vi "ScratchImage.vi"() -> ()   [LabVIEW 2020]
uses:
  <vilib>/Analysis/baseanly.llb/Mean (DBL).vi
  <vilib>/Analysis/NI_AALBase.lvlib
panel:
  in  "Save to Files":bool
  in  "Path":path
  out "height":dbl
  out "width":dbl
  out "y":dbl format="%0.2f"
  out "x":dbl format="%0.2f"
  out "new picture":picture
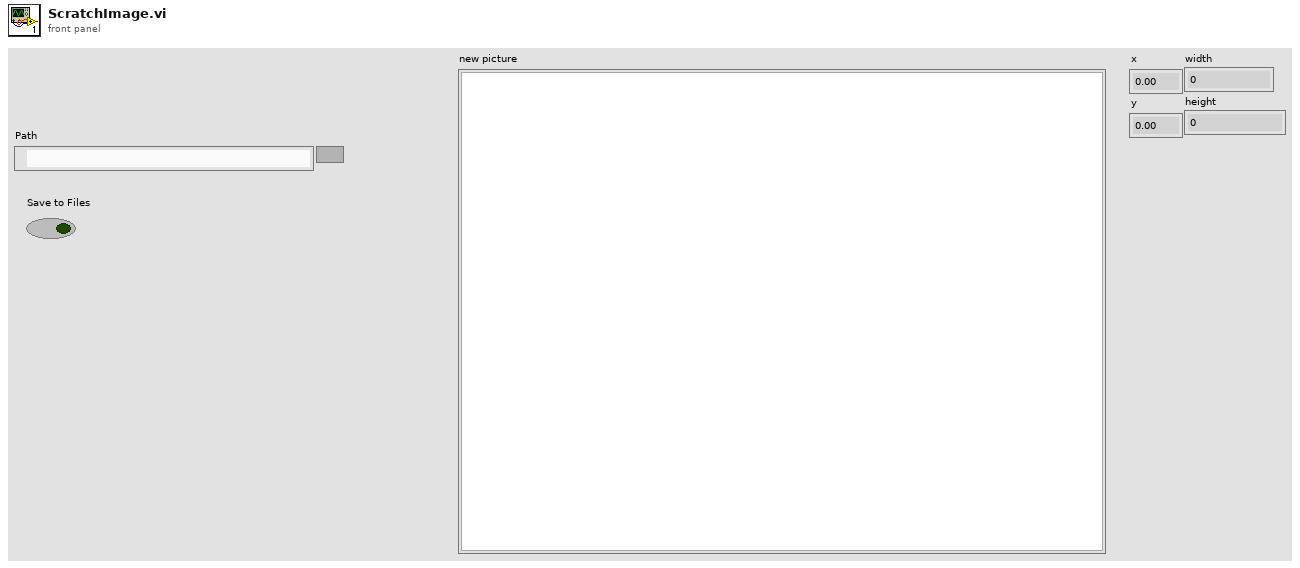
[diagram p1: front panel]
types:
  T1 = enum16{"open", "replace", "create", "open or create", "replace or create", "replace or create with confirmation"}
  T2 = cluster{"Width":u16, "Style":enum32{"Solid", "Dash", "Dot", "DashDot", "DashDotDot"}}
  T3 = enum32{"Solid", "Dash", "Dot", "DashDot", "DashDotDot"}
  T4 = typedef "imagedata.ctl" = cluster{"image type":i32, "image depth":i32, "image":u8[], "mask":u8[], "colors":u32[], "Rectangle":cluster{"left":i16, "top":i16, "right":i16, "bottom":i16}}
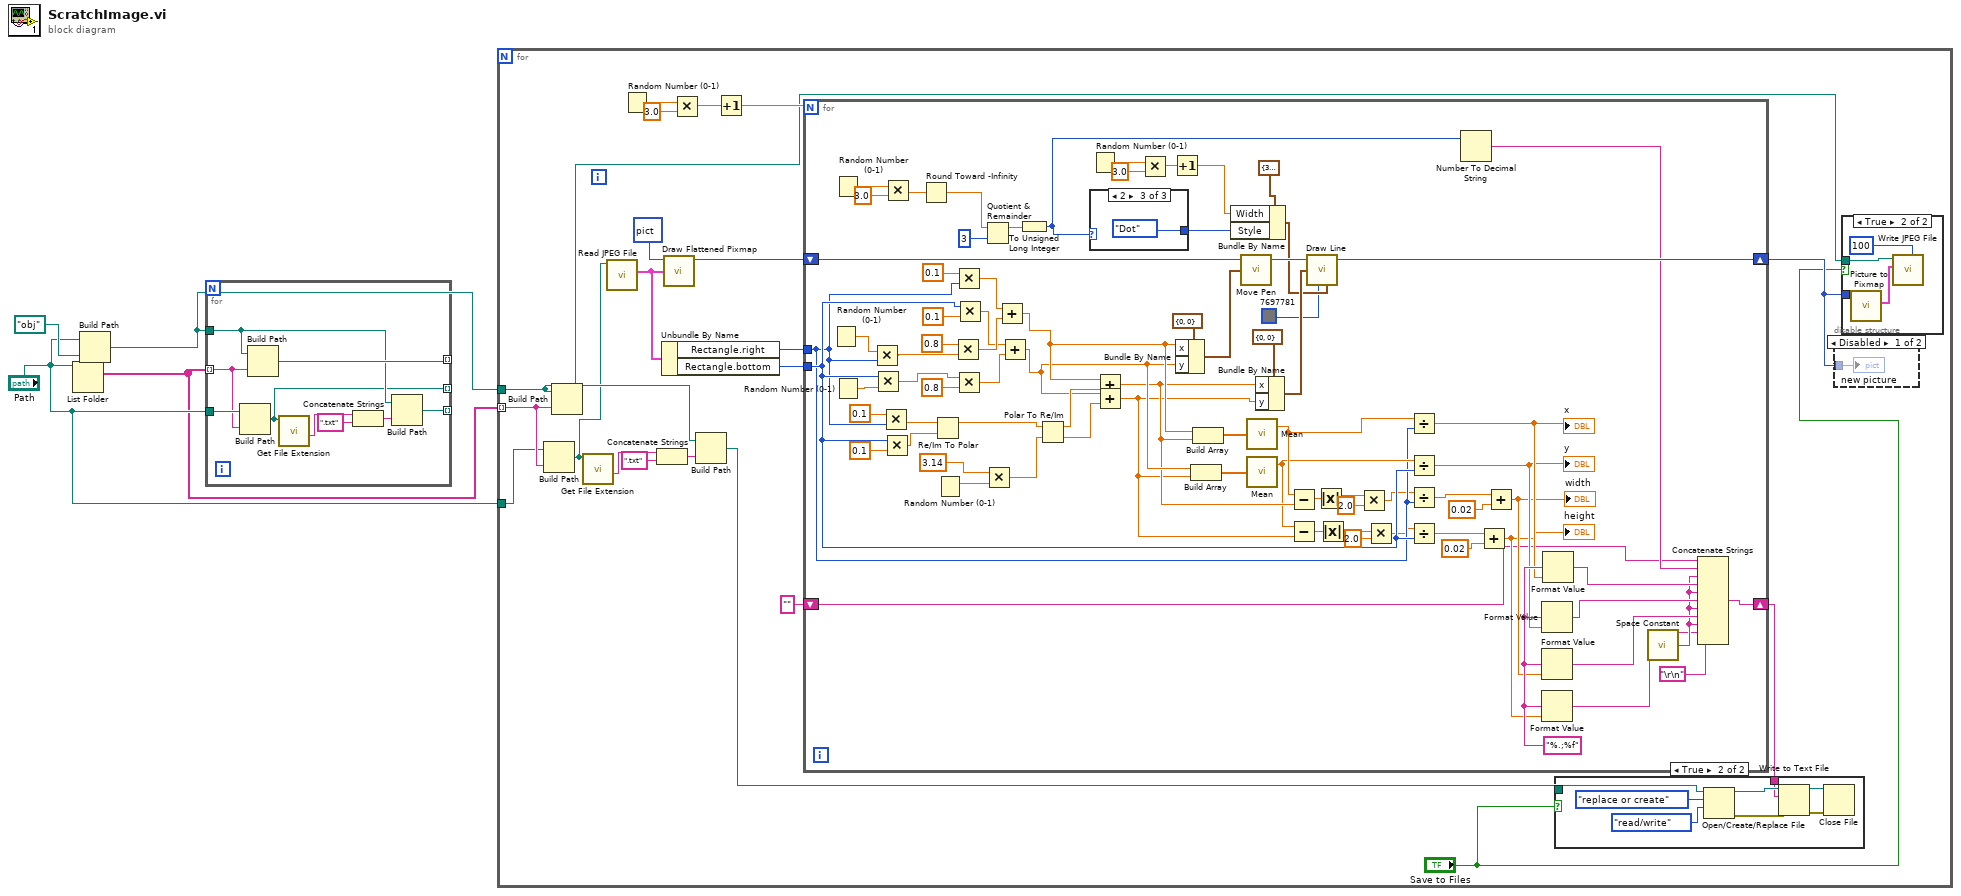
[diagram p0: block diagram]
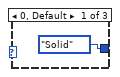
[diagram p5: hidden frame]
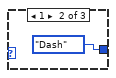
[diagram p6: hidden frame]
diagram:
  n1 = List Folder(path="Path") -> (filenames=w1:string[])  [unwired: 3 in, 3 out]
  n2 = Build Path(base path="Path", name or relative path=path "obj") -> (appended path=w3:path)
  n3 = for {
    tunnel: w1 -> [w11] mode=indexing
    tunnel: w3 -> [w10]
    tunnel: [w13] -> _ mode=indexing
    tunnel: "Path" -> [w12]
    tunnel: [w6] -> _ mode=indexing
    tunnel: [w5] -> _ mode=indexing
    n4 = Build Path(base path=w12, name or relative path=w11) -> (appended path=w5:path)
    n5 = Build Path(base path=w10, name or relative path=w11) -> (appended path=w13:path)
    n6 = call <vilib>:"Get File Extension.vi"("file"=w5) -> ("filename without extension"=w8:string)  [unwired: 6 in, 4 out]
    n7 = Concatenate Strings(w8, ".txt" ("string")) -> (w9:string)
    n8 = Build Path(base path=w10, name or relative path=w9) -> (appended path=w6:path)
  }
  n9 = for {
    tunnel: w3 -> [w26]
    tunnel: w1 -> [w25] mode=indexing
    tunnel: "Path" -> [w24]
    n10 = Build Path(base path=w24, name or relative path=w25) -> (appended path=w22:path)
    n11 = Build Path(base path=w26, name or relative path=w25) -> (appended path=w17:path)
    n12 = call <vilib>:"Get File Extension.vi"("file"=w22) -> ("filename without extension"=w28:string)  [unwired: 6 in, 4 out]
    n13 = call <vilib>:"Read JPEG File.vi"("path to JPEG file"=w22) -> ("image data"=w33:T4)  [unwired: 8 in, 2 out]
    n14 = Random Number (0-1)() -> (number: 0 to 1=w21:dbl)
    n15 = Concatenate Strings(w28, ".txt" ("string")) -> (w29:string)
    n16 = Unbundle By Name(w33) -> ("Rectangle.right"=w31:i16, "Rectangle.bottom"=w32:i16)
    n17 = call <vilib>:"Draw Flattened Pixmap.vi"("image data"=w33, "picture"=picture data[5B]) -> ("new picture"=w34:picture)  [unwired: 7 in]
    n18 = Multiply(x=w21, y=3.0) -> (x*y=w19:dbl)
    n19 = Build Path(base path=w26, name or relative path=w29) -> (appended path=w23:path)
    n20 = Increment(x=w19) -> (x+1=w18:dbl)
    n21 = for {
      N: w18 -> [_]
      tunnel: w32 -> [w85]
      tunnel: w31 -> [w84]
      shift-right: [w61] -> w16
      shift-left: w34 -> [w128]
      shift-right: [w70] -> w30
      shift-left: "" -> [w49]
      w72 = "%.;%f" ("format string")
      n22 = Random Number (0-1)() -> (number: 0 to 1=w124:dbl)
      n23 = Random Number (0-1)() -> (number: 0 to 1=w56:dbl)
      n24 = Random Number (0-1)() -> (number: 0 to 1=w125:dbl)
      n25 = Multiply(x=w124, y=w84) -> (x*y=w108:dbl)
      n26 = Multiply(x=w85, y=w125) -> (x*y=w107:dbl)
      n27 = Multiply(x=0.1 ("y"), y=w84) -> (x*y=w120:dbl)
      n28 = Multiply(x=w85, y=0.1) -> (x*y=w119:dbl)
      n29 = Multiply(x=w56, y=3.0) -> (x*y=w54:dbl)
      n30 = Round Toward -Infinity(1:w54) -> (0:w53:dbl)
      n31 = Re/Im To Polar(2:w119, 3:w120) -> (1:w116:dbl)  [unwired: 1 out]
      n32 = Random Number (0-1)() -> (number: 0 to 1=w118:dbl)
      n33 = Multiply(x=0.8 ("y"), y=w108) -> (x*y=w102:dbl)
      n34 = Multiply(x=0.1 ("y"), y=w84) -> (x*y=w104:dbl)
      n35 = Multiply(x=w107, y=0.8) -> (x*y=w103:dbl)
      n36 = Multiply(x=w85, y=0.1) -> (x*y=w101:dbl)
      n37 = Quotient & Remainder(x=w53, y=3) -> (x-y*floor(x/y)=w52:dbl)  [unwired: 1 out]
      n38 = Multiply(x=3.14, y=w118) -> (x*y=w115:dbl)
      n39 = Add(x=w104, y=w102) -> (x+y=w95:dbl)
      n40 = Add(x=w101, y=w103) -> (x+y=w94:dbl)
      n41 = To Unsigned Long Integer(number=w52) -> (unsigned 32bit integer=w51:u32)
      n42 = Polar To Re/Im(2:w115, 3:w116) -> (0:w114:dbl, 1:w113:dbl)
      n43 = Random Number (0-1)() -> (number: 0 to 1=w60:dbl)
      n44 = case shown="2" w51 {
        tunnel: [T3."Solid" ("Style") T3."Dash" ("Style") T3."Dot" ("Style")] -> w96
        frame 0, Default {
        }
        frame 1 {
        }
        frame 2 {
        }
      }
      n45 = Add(x=w95, y=w113) -> (x+y=w91:dbl)
      n46 = Add(x=w94, y=w114) -> (x+y=w90:dbl)
      n47 = Multiply(x=w60, y=3.0) -> (x*y=w58:dbl)
      n48 = Increment(x=w58) -> (x+1=w57:dbl)
      n49 = Bundle By Name(cluster=cluster{"x":i16, "y":i16} {"x"=0, "y"=0} ("new position"), "x"=w95, "y"=w94) -> (w123:cluster{"x":i16, "y":i16})
      n50 = Build Array(w94, w90) -> (w92:dbl[])
      n51 = Build Array(w95, w91) -> (w93:dbl[])
      n52 = Bundle By Name(cluster=T2 {"Width"=3, "Style"=enum."Dot"} ("pen"), "Width"=w57, "Style"=w96) -> (w98:T2)
      n53 = call <vilib>:"Move Pen.vi"("new position"=w123, "picture"=w128) -> ("new picture"=w127:picture)  [unwired: 3 in]
      n54 = call-poly <vilib>:"Mean.vi"("X"=w93) -> ("mean"=w87:dbl)  [unwired: 1 out]
      n55 = call-poly <vilib>:"Mean.vi"("X"=w92) -> ("mean"=w86:dbl)  [unwired: 1 out]
      n56 = Bundle By Name(cluster=cluster{"x":i16, "y":i16} {"x"=0, "y"=0} ("new position"), "x"=w91, "y"=w90) -> (w111:cluster{"x":i16, "y":i16})
      n57 = Subtract(x=w87, y=w91) -> (x-y=w89:dbl)
      n58 = Subtract(x=w86, y=w90) -> (x-y=w88:dbl)
      n59 = call <vilib>:"Draw Line.vi"("picture"=w127, "end point"=w111, "color(black)"=u32 7697781, "pen"=w98) -> ("new picture"=w61:picture)  [unwired: 5 in]
      n60 = Absolute Value(x=w89) -> (abs(x)=w83:dbl)
      n61 = Absolute Value(x=w88) -> (abs(x)=w79:dbl)
      n62 = Multiply(x=w83, y=2.0) -> (x*y=w80:dbl)
      n63 = Multiply(x=w79, y=2.0) -> (x*y=w78:dbl)
      n64 = Divide(x=w87, y=w84) -> (x/y=w69:dbl)
      "x" <- w69
      n65 = Divide(x=w86, y=w85) -> (x/y=w64:dbl)
      "y" <- w64
      n66 = Divide(x=w80, y=w84) -> (x/y=w65:dbl)
      n67 = Divide(x=w78, y=w85) -> (x/y=w66:dbl)
      n68 = Number To Decimal String(number=w51) -> (decimal integer string=w50:string)  [unwired: 1 in]
      n69 = Add(x=w66, y=0.02) -> (x+y=w62:dbl)
      "height" <- w62
      n70 = Add(x=w65, y=0.02) -> (x+y=w63:dbl)
      "width" <- w63
      n71 = Format Value(format string=w72, value (0)=w64) -> (output string=w76:string)  [unwired: 1 in]
      n72 = Format Value(format string=w72, value (0)=w63) -> (output string=w75:string)  [unwired: 1 in]
      n73 = Format Value(format string=w72, value (0)=w62) -> (output string=w71:string)  [unwired: 1 in]
      n74 = Format Value(format string=w72, value (0)=w69) -> (output string=w77:string)  [unwired: 1 in]
      n75 = call <vilib>:"Space Constant.vi"() -> ("String"=w73:string)
      n76 = Concatenate Strings(w49, w50, w73, w77, w73, w76, w73, w75, w73, w71, "\r\n") -> (w70:string)
    }
    n77 = case shown="True" "Save to Files" {
      tunnel: w30 -> [_ w42]
      tunnel: w23 -> [_ w41]
      frame False {
      }
      frame True {
        n78 = Open/Create/Replace File(file path (use dialog)=w41, operation (0:open)=T1."replace or create", access (0:read/write)=enum16{"read/write", "read-only", "write-only"}."read/write") -> (refnum out=w45:refnum<file>, error out=w44:errorcluster)  [unwired: 3 in, 1 out]
        n79 = Write to Text File(file (use dialog)=w45, text=w42, error in=w44) -> (refnum out=w48:refnum<file>, error out=w47:errorcluster)  [unwired: 1 in, 1 out]
        n80 = Close File(refnum=w48, error in=w47) -> ()  [unwired: 2 out]
      }
    }
    n81 = disable-structure shown="Disabled" {
      disable-tunnel: w16 -> [w36 _]
      frame Disabled {
        "new picture" <- w36
      }
      frame Enabled {
      }
    }
    n82 = case shown="True" "Save to Files" {
      tunnel: w17 -> [_ w38]
      tunnel: w16 -> [_ w37]
      frame False {
      }
      frame True {
        n83 = call <vilib>:"Picture to Pixmap.vi"("picture"=w37) -> ("image data"=w40:T4)  [unwired: 9 in, 1 out]
        n84 = call <vilib>:"Write JPEG File.vi"("quality (80)"=100, "image data"=w40, "path to JPEG file"=w38) -> ()  [unwired: 7 in, 2 out]
      }
    }
  }
